vi "lsi_finetune.vi"(6 "timeout (25000ms)":i32=25000, 8 "error in (no error)":errorcluster, 10 "parameter":T1={"speed in rpm"=0.0, "Delta_tmag_lsi_degC"=0.0, "Delta_tmag_%"=100.0}, 11 "daemon reference in":refnum<k5>) -> (0 "error out":errorcluster, 2 "response":string, 3 "daemon reference out":refnum<k5>, 5 "command out":string="random")   [LabVIEW 2017]
doc: "<b>Command: </b>\"lsi_finetune\"\n\n<b>Description: </b> This command performs an lsi fine tune constant for eol_bemf_lsi_mp_coeff_c\n\n<b>Parameters: </b> speed in rpm, delta_tmag -signed temperature delta, delta_tmag_percent - percentage level signed deltag \n____________________________________________\nDIPC 692 Daemon API 10.0.0.1\nSam Tee - Dyson Technology Ltd\nCopyright (c) 2024, Dyson Technology Ltd"
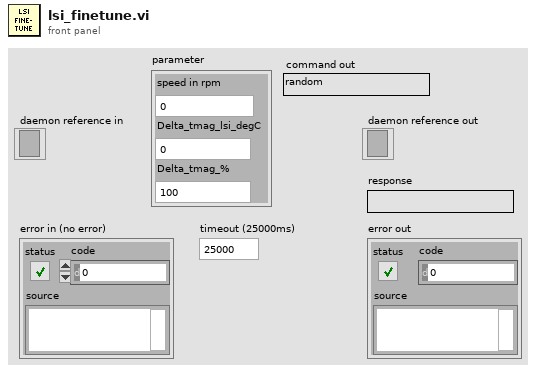
[diagram p1: front panel]
types:
  T1 = cluster{"speed in rpm":dbl, "Delta_tmag_lsi_degC":dbl, "Delta_tmag_%":dbl}
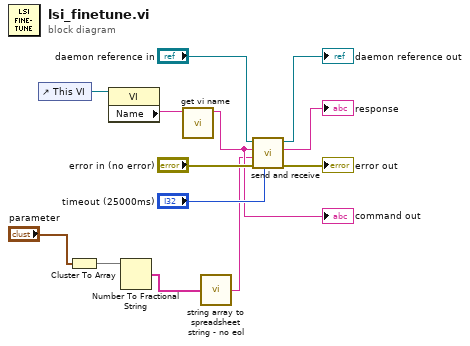
[diagram p0: block diagram]
diagram:
  n1 = control-ref of="This VI"() -> (w7:refnum<vi>)
  n2 = Cluster To Array(cluster="parameter") -> (array=w3:dbl[])
  n3 = property class="VI"(reference=w7) -> ("Name"=w6:string)  [unwired: 1 in, 2 out]
  n4 = Number To Fractional String(number=w3) -> (F-format string=w2:string[])  [unwired: 3 in]
  n5 = call "get vi name.vi"("library.lvlib:name.vi"=w6) -> ("vi name"=w5:string)  [unwired: 10 in]
  "command out" <- w5
  n6 = call "string array to spreadsheet string - no eol.vi"("string array"=w2) -> ("spreadsheet string - no eol"=w1:string)
  n7 = call "send and receive.vi"("timeout (25000ms)"="timeout (25000ms)", "error in (no error)"="error in (no error)", "data"=w1, "command"=w5, "daemon reference in"="daemon reference in") -> ("error out"=→"error out":errorcluster, "response"=→"response":string, "daemon reference out"=→"daemon reference out":refnum<k5>)  [unwired: 4 in]
